vi "Test GPS Signal.vi"(8 "STOP PROGRAM":bool, 11 "VISA resource name":refnum<visa-resource-name>="COM4") -> ()   [LabVIEW 2011]
panel:
  out "GPS Initialize Error":errorcluster
  out "Read Buffer":string
  out "Latitude":dbl format="%_11g"
  out "Longitude":dbl format="%_12g"
  out "Altitude Above Mean Sea Level (m)":string
  out "Satellites Tracked":string
  out "Fixed Quality":string
  out "East or West":string
  out "North or South":string
  out "Sample Time":string
  out "GPS Acquire Error":errorcluster
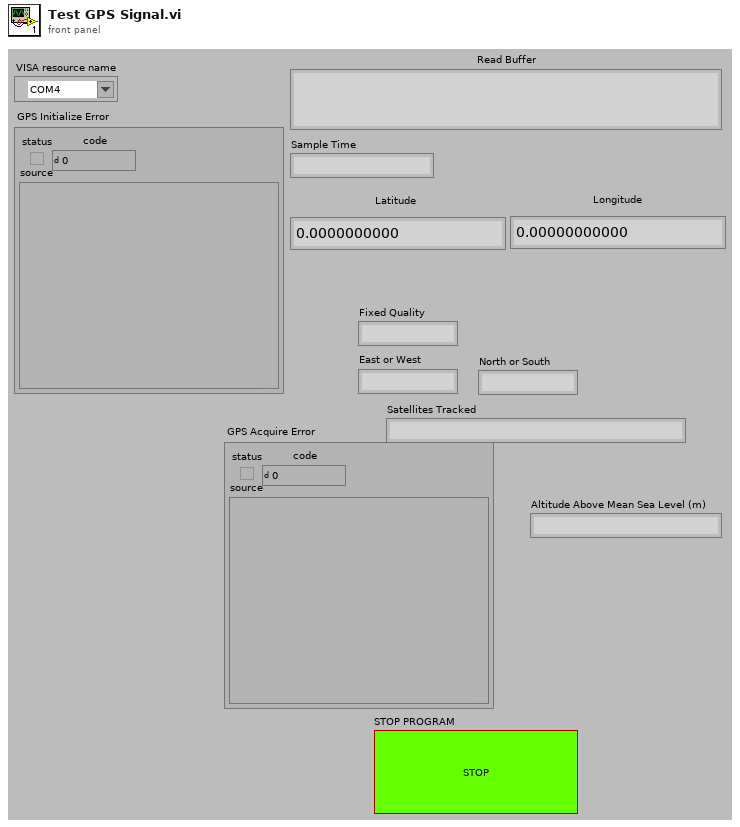
[diagram p1: front panel]
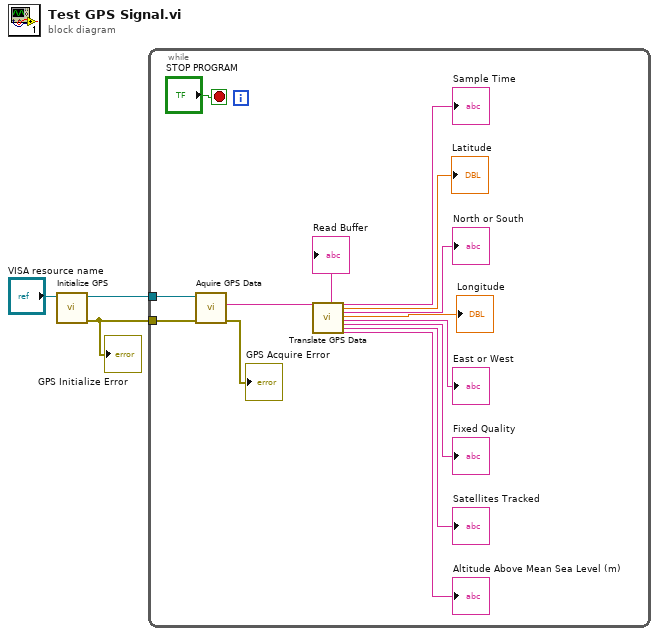
[diagram p0: block diagram]
diagram:
  n1 = call "Initialize GPS.vi"("VISA resource name"="VISA resource name") -> ("error out"=w1:errorcluster, "VISA resource name out"=w2:refnum<visa-resource-name>)  [unwired: 9 in]
  "GPS Initialize Error" <- w1
  n2 = while {
    tunnel: w1 -> [w13]
    tunnel: w2 -> [w12]
    stop <- "STOP PROGRAM" stop-if-true
    n3 = call "Aquire GPS Data.vi"("error in"=w13, "VISA resource name in"=w12) -> ("error out"=→"GPS Acquire Error":errorcluster, "read buffer"=w4:string)  [unwired: 7 in, 1 out]
    "Read Buffer" <- w4
    n4 = call "Translate GPS Data.vi"("Read Buffer"=w4) -> ("Sample Time"=→"Sample Time":string, "Latitude"=→"Latitude":dbl, "North or South"=→"North or South":string, "Longitude"=→"Longitude":dbl, "East or West"=→"East or West":string, "Fixed Quality"=→"Fixed Quality":string, "Satellites Tracked"=→"Satellites Tracked":string, "Altitude Above Mean Sea Level (m)"=→"Altitude Above Mean Sea Level (m)":string)  [unwired: 19 in]
  }
